vi "Quik Stop Motors.vi"(7 "timeout (1s)":dbl=1.0 min=0.0, 8 "error in (no error)":errorcluster, 9 "Left motor Clustered SDO":T1, 10 "Right motor Clustered SDO":T1, 11 "CANOpen session":refnum<k20>) -> (0 "error out":errorcluster, 1 "completion code":u32, 3 "CANOpen session":refnum<k20>)   [LabVIEW 2016]
uses:
  RT/Clustered SDO.ctl
  RT/Set Controlword.vi
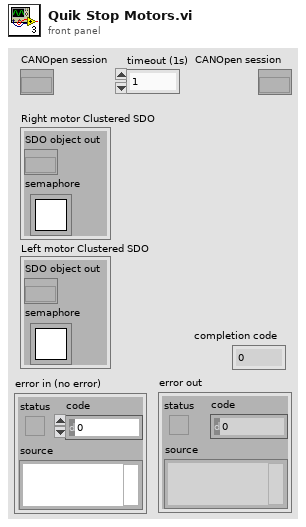
[diagram p1: front panel]
types:
  T1 = typedef "Clustered SDO.ctl" = cluster{"SDO object out":refnum<k20>, "semaphore":T2}
  T2 = typedef "Semaphore RefNum" = refnum<k1>
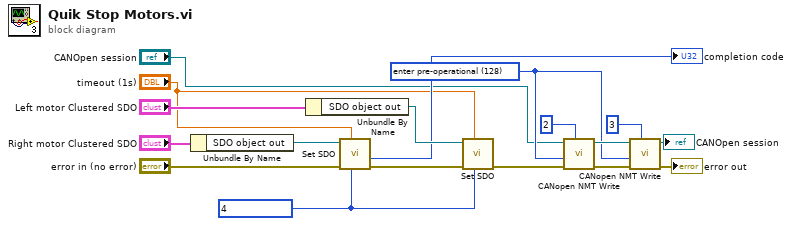
[diagram p0: block diagram]
diagram:
  w14 = u8 4 ("Controlword")
  w9 = u16 128 items=["start remote node"=1, "stop remote node"=2, "enter pre-operational"=128, "reset node"=129, "reset communication"=130] ("command")
  n1 = Unbundle By Name("Right motor Clustered SDO") -> ("SDO object out"=w17:refnum<k20>)
  n2 = Unbundle By Name("Left motor Clustered SDO") -> ("SDO object out"=w16:refnum<k20>)
  n3 = call-poly "Set SDO.vi"("Controlword"=w14, "timeout (1s)"="timeout (1s)", "error in (no error)"="error in (no error)", "SDO object in"=w17) -> ("error out"=w13:errorcluster, "completion code"=→"completion code":u32)  [unwired: 5 in, 1 out]
  n4 = call-poly "Set SDO.vi"("Controlword"=w14, "timeout (1s)"="timeout (1s)", "error in (no error)"=w13, "SDO object in"=w16) -> ("error out"=w12:errorcluster)  [unwired: 5 in, 2 out]
  n5 = call <vilib>:"CANopen NMT Write.vi"("node-ID (0)"=u8 2, "error in (no error)"=w12, "command"=w9, "interface object in"="CANOpen session") -> ("error out"=w11:errorcluster, "interface object out"=w10:refnum<k20>)  [unwired: 6 in]
  n6 = call <vilib>:"CANopen NMT Write.vi"("node-ID (0)"=u8 3, "error in (no error)"=w11, "command"=w9, "interface object in"=w10) -> ("error out"=→"error out":errorcluster, "interface object out"=→"CANOpen session":refnum<k20>)  [unwired: 6 in]
